vi "AuMT8852B EDR Sensitivity Configuration.vi"(5 "Settings":T2={"Low frequency selection"=enum."Use low frequency", "Medium frequency selection"=enum."Use medium frequency", "High frequency selection"=enum."Use high frequency", "Low TX frequency"=2480.0, "Low RX frequency"=2402.0, "Medium TX frequency"=2402.0, "Medium RX frequency"=2441.0, "High TX frequency"=2402.0, "High RX frequency"=2480.0, "Threshold bit count"=0.1, "2DHx test packet"=enum."OFF", "3DHx test packet"=enum."OFF", "Hop selection"=enum."Test with hopping off and on", "Test TX power"=-70.0, "Packet count"=enum."TX", "Total test bit count"=0.1, "Use Dirty transmitter"=FALSE, "Symbol timing error (ppm)"=[-20, -20, 20, 20, 20, -20, -20, -20, -20, 20], "Frequency offset (kHz)"=[75.0, 14.0, -2.0, 1.0, 39.0, 0.0, -42.0, 74.0, -19.0, -75.0], "Threshold error limit (E-5)"=7, "Total test error limit (E-4)"=1} {"Frequency offset (kHz)" format="%.2f"; "Symbol timing error (ppm)" format="%.1f"; "Total test bit count" format="%.2f"; "Test TX power" format="%.1f"; "Threshold bit count" format="%.2f"}, 7 "Set/Get (Set)":enum16{"Set", "Get"}(ring), 8 "error in (no error)":errorcluster, 10 "Script (3)":i32=3, 11 "VISA session":refnum<visa-resource-name>) -> (0 "error out":errorcluster, 2 "error code":i32, 3 "VISA session out":refnum<visa-resource-name>, 4 "Settings out":T1={"Low frequency selection"=enum."Use low frequency", "Medium frequency selection"=enum."Use medium frequency", "High frequency selection"=enum."Use high frequency", "Low TX frequency"=2480.0, "Low RX frequency"=2402.0, "Medium TX frequency"=2402.0, "Medium RX frequency"=2441.0, "High TX frequency"=2402.0, "High RX frequency"=2480.0, "Threshold bit count"=0.1, "2DHx test packet"=enum."OFF", "3DHx test packet"=enum."OFF", "Hop selection"=enum."Test with hopping off and on", "Test TX power"=-70.0, "Packet count"=enum."TX", "Total test bit count"=0.1, "Use Dirty transmitter"=FALSE, "Symbol timing error (ppm)"=[-20.0, -20.0, 20.0, 20.0, 20.0, -20.0, -20.0, -20.0, -20.0, 20.0], "Frequency offset (kHz)"=[75.0, 14.0, -2.0, 1.0, 39.0, 0.0, -42.0, 74.0, -19.0, -75.0], "Threshold error limit (E-5)"=7, "Total test error limit (E-4)"=1} {"Frequency offset (kHz)" format="%.2f"; "Symbol timing error (ppm)" format="%.2f"; "Total test bit count" format="%.2f"; "Test TX power" format="%.1f"; "Threshold bit count" format="%.2f"})   [LabVIEW 2017]
doc: "Anritsu MT8852B Bluetooth Tester\n\nConfigures the instrument for the EDR Sensitivity test.\n\nINPUTS\nSet/Get - whether the values are being sent to or retrieved from the instrument.\nScript - which of the stored scripts (1-10) will be queried or configured. Scripts 1 and 2 are read-only.\nSettings - parameters of the test to be written.\n\nOUTPUTS\nSettings out - current parameters of the test."
uses:
  <instrlib>/aumt8852B/General/Utilities/MT8850 Test Parameters.ctl
  <instrlib>/aumt8852B/General/Utilities/MT8850 Frequency Units.ctl
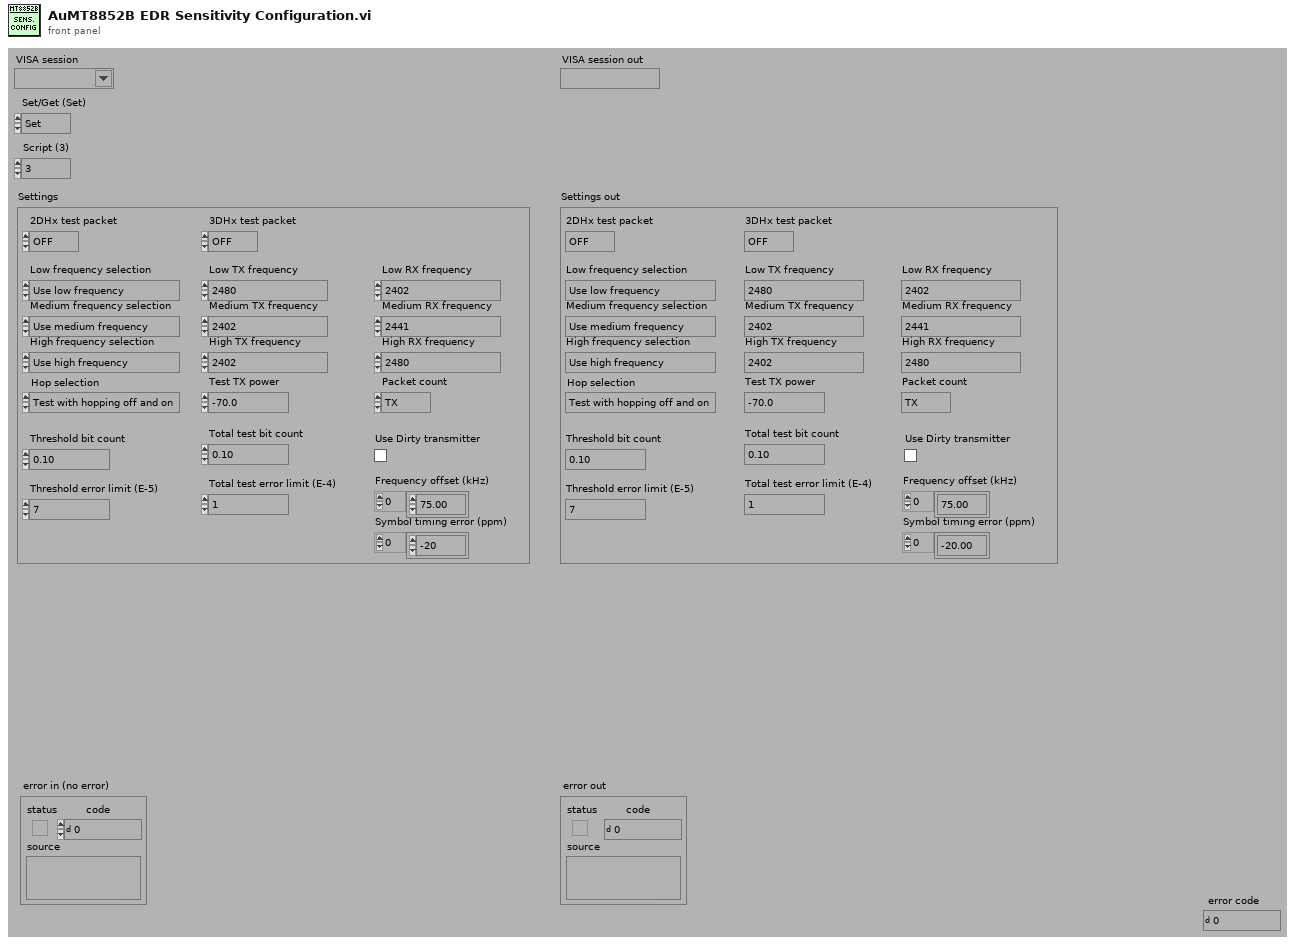
[diagram p1: front panel]
types:
  T1 = cluster{"Low frequency selection":enum16{"Don't use low frequency", "Use low frequency"}, "Medium frequency selection":enum16{"Don't use medium frequency", "Use medium frequency"}, "High frequency selection":enum16{"Don't use high frequency", "Use high frequency"}, "Low TX frequency":dbl, "Low RX frequency":dbl, "Medium TX frequency":dbl, "Medium RX frequency":dbl, "High TX frequency":dbl, "High RX frequency":dbl, "Threshold bit count":dbl, "2DHx test packet":enum16{"OFF", "Longest", "2-DH1", "2-DH3", "2-DH5"}, "3DHx test packet":enum16{"OFF", "Longest", "3-DH1", "3-DH3", "3-DH5"}, "Hop selection":enum16{"Test with hopping on", "Test with hopping off", "Test with hopping off and on"}, "Test TX power":dbl, "Packet count":enum16{"TX", "RX"}, "Total test bit count":dbl, "Use Dirty transmitter":bool, "Symbol timing error (ppm)":dbl[], "Frequency offset (kHz)":dbl[], "Threshold error limit (E-5)":i16, "Total test error limit (E-4)":i16}
  T2 = cluster{"Low frequency selection":enum16{"Don't use low frequency", "Use low frequency"}, "Medium frequency selection":enum16{"Don't use medium frequency", "Use medium frequency"}, "High frequency selection":enum16{"Don't use high frequency", "Use high frequency"}, "Low TX frequency":dbl, "Low RX frequency":dbl, "Medium TX frequency":dbl, "Medium RX frequency":dbl, "High TX frequency":dbl, "High RX frequency":dbl, "Threshold bit count":dbl, "2DHx test packet":enum16{"OFF", "Longest", "2-DH1", "2-DH3", "2-DH5"}, "3DHx test packet":enum16{"OFF", "Longest", "3-DH1", "3-DH3", "3-DH5"}, "Hop selection":enum16{"Test with hopping on", "Test with hopping off", "Test with hopping off and on"}, "Test TX power":dbl, "Packet count":enum16{"TX", "RX"}, "Total test bit count":dbl, "Use Dirty transmitter":bool, "Symbol timing error (ppm)":i8[], "Frequency offset (kHz)":dbl[], "Threshold error limit (E-5)":i16, "Total test error limit (E-4)":i16}
  T3 = enum16{"Frequency offset", "Symbol timing value", "Mod index value"}
  T4 = enum16{"Single-slot sensitivity", "Multiple-slot sensitivity", "EDR sensitivity"}
  T5 = typedef "MT8850 Test Parameters.ctl" = enum16{"Use low frequency", "Use medium frequency", "Use high frequency", "Low TX frequency", "Low RX frquency", "Medium TX frequency", "Medium RX frequency", "High TX frequency", "High RX frequency", "Number of packets", "Average high limit", "Average low limit", "Peak power limit", "Max power step limit", "Min power step limit", "f1 average minimum", "f1 average maximum", "f2 maximum", "f1/f2 average maximum", "Hop selection", "Use DH1 packets", "Use DH3 packets", "Use DH5 packets", "1 slot packet drift limit", "3 slot packet drift limit", "5 slot packet drift limit", "Drift rate limit", "TX power level", "Frequency offset", "Symbol timing", "Modulation index", "BER limit", "FER limit", "Use averaging high limit", "Use averaging low limit", "Use peak power limit", "Packet type", "Test control", "Use max power step limit", "Use min power step limit", "Number of cycles", "Use f1 average maximum", "Use f1 average minimum", "Use f2 maximum", "Use f1/f2 average maximum", "Hop mode", "Maximum negative limit", "Maximum positive limit", "Use maximum negative limit", "Use maximum positive limit", "Use 1 slot packet drift limit", "Use 3 slot packet drift limit", "Use 5 slot packet drift limit", "Use drift rate limit", "Use BER limit", "Use FER limit", "Use dirty parameter table", "Use null packet drift limit", "Null packet drift limit", "Minimum power", "Power delay", "Packet count", "Payload toggle", "Output power level", "2DHX packet type", "3DHX packet type", "Number of blocks", "TX and RX low frequency", "TX and RX medium frequency", "TX and RX high frequency", "TX frequency", "RX frequency", "Threshold bit count", "Total test bit count", "Number of bits", "PDPSK to PGFSK lower limit", "PDPSK to PGFSK upper limit", "Initial frequency error upper limit", "Initial frequency error lower limit", "Frequency error upper limit", "Frequency error lower limit", "Block frequency error upper limit", "Block frequency error lower limit", "2Mbs RMS DEVM limit", "3Mbs RMS DEVM limit", "2Mbs Peak DEVM limit", "3Mbs Peak DEVM limit", "2Mbs 99% packets DEVM limit", "3Mbs 99% packets DEVM limit", "Percentage of no error packets limit", "Threshold error limit", "Total test error limit"}
  T6 = enum16{"Output power", "Power control", "Modulation characteristics", "Initial carrier", "Carrier drift", "Single slot sensitivity", "Multiple slot sensitivity", "Maximum input power", "EDR Relative transmit power", "EDR Carrier frequency and stability", "EDR Differential phase encoding", "EDR Sensitivity", "EDR BER floor sensitivity", "EDR Maximum input power"}
  T7 = typedef "MT8850 Frequency Units.ctl" = enum16{"Channel", "Hz", "kHz", "MHz", "GHz"}
  T8 = enum16{"Simulate", "Range check", "Cache", "Query instrument status"}
  T9 = enum16{"Test with hopping on", "Test with hopping off", "Test with hopping off and on"}
  T10 = enum16{"OFF", "Longest", "3-DH1", "3-DH3", "3-DH5"}
  T11 = enum16{"OFF", "Longest", "2-DH1", "2-DH3", "2-DH5"}
  T12 = enum16{"Don't use high frequency", "Use high frequency"}
  T13 = enum16{"Don't use medium frequency", "Use medium frequency"}
  T14 = enum16{"Don't use low frequency", "Use low frequency"}
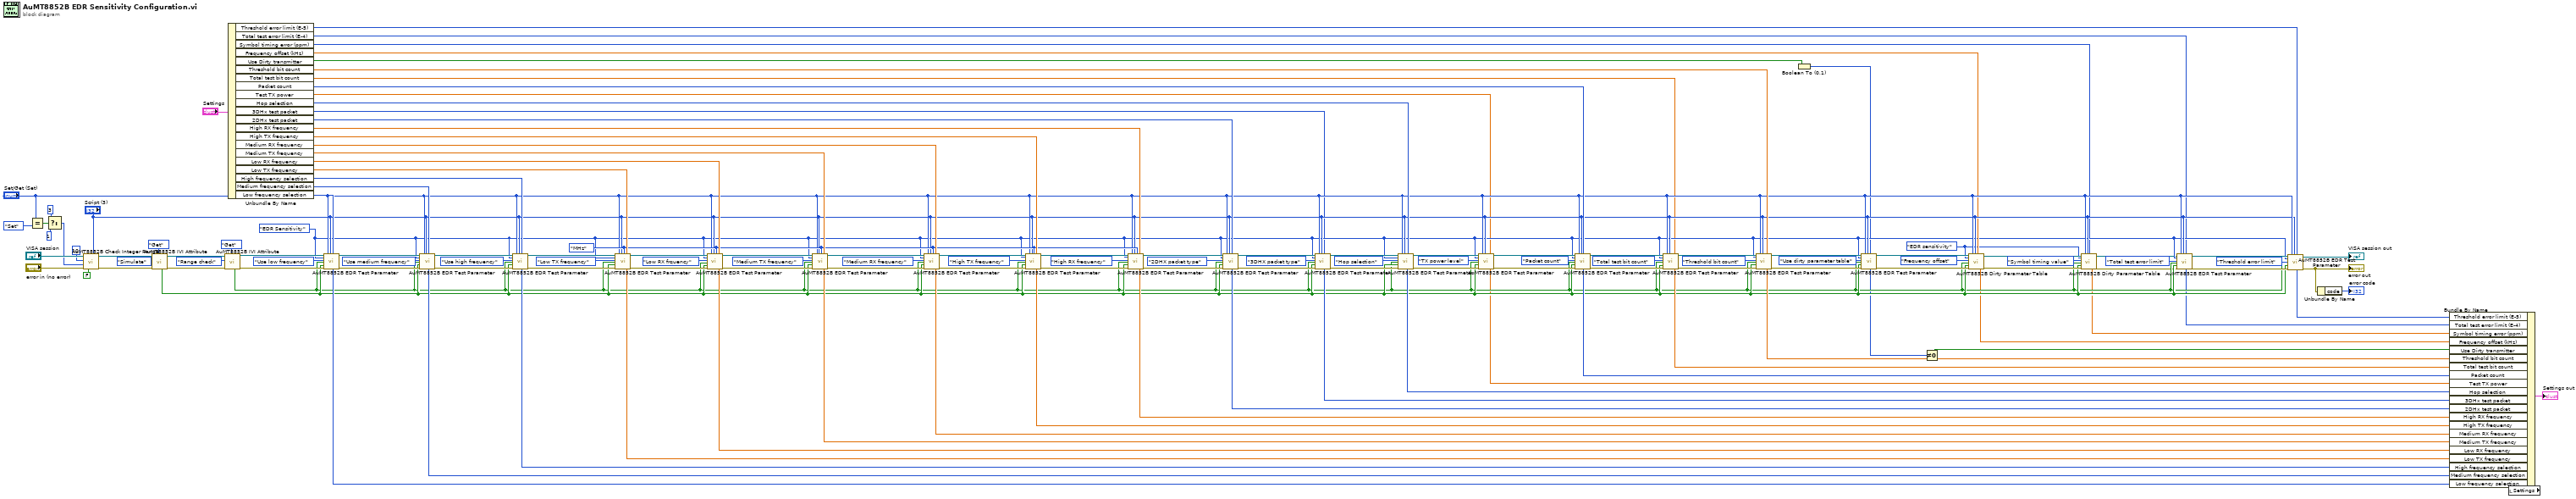
[diagram p0: block diagram]
diagram:
  w14 = T4."EDR sensitivity" ("Test (Single-slot sensitivity)")
  w15 = T6."EDR Sensitivity" ("Test (Output power)")
  w65 = MT8850_Frequency_Units."MHz" ("Frequency units (MHz)")
  n1 = Equal?(x="Set/Get (Set)", y=enum16{"Set", "Get"}."Set") -> (x = y?=w134:bool)
  n2 = Select(t=3, s=w134, f=1) -> (s? t:f=w130:i32)
  n3 = call <instrlib>:"AuMT8852B Check Integer Range.vi"("Value (0)"="Script (3)", "Check IVI flag first? (T)"=FALSE, "error in (no error)"="error in (no error)", "Lower limit (-1)"=w130, "Upper limit (1)"=10, "VISA session"="VISA session") -> ("error out"=w128:errorcluster, "VISA session out"=w129:refnum<visa-resource-name>)  [unwired: 4 in]
  n4 = call <instrlib>:"AuMT8852B IVI Attribute.vi"("Set/Get (Set)"=enum16{"Set", "Get"}."Get", "error in (no error)"=w128, "Flag (Simulate)"=T8."Simulate", "VISA session"=w129) -> ("error out"=w102:errorcluster, "VISA session out"=w103:refnum<visa-resource-name>, "Value out"=w30:bool)  [unwired: 5 in]
  n5 = call <instrlib>:"AuMT8852B IVI Attribute.vi"("Set/Get (Set)"=enum16{"Set", "Get"}."Get", "error in (no error)"=w102, "Flag (Simulate)"=T8."Range check", "VISA session"=w103) -> ("error out"=w100:errorcluster, "VISA session out"=w101:refnum<visa-resource-name>, "Value out"=w29:bool)  [unwired: 5 in]
  n6 = Unbundle By Name("Settings") -> ("Threshold error limit (E-5)"=w2:i16, "Total test error limit (E-4)"=w3:i16, "Symbol timing error (ppm)"=w11:i8[], "Frequency offset (kHz)"=w17:dbl[], "Use Dirty transmitter"=w19:bool, "Threshold bit count"=w35:dbl, "Total test bit count"=w7:dbl, "Packet count"=w50:enum16{"TX", "RX"}, "Test TX power"=w1:dbl, "Hop selection"=w56:T9, "3DHx test packet"=w8:T10, "2DHx test packet"=w78:T11, "High RX frequency"=w90:dbl, "High TX frequency"=w91:dbl, "Medium RX frequency"=w79:dbl, "Medium TX frequency"=w92:dbl, "Low RX frequency"=w93:dbl, "Low TX frequency"=w94:dbl, "High frequency selection"=w95:T12, "Medium frequency selection"=w96:T13, "Low frequency selection"=w97:T14)
  n7 = call <instrlib>:"AuMT8852B EDR Test Parameter.vi"("VISA session"=w101, "Test (Output power)"=w15, "Parameter (Use low frequency)"=MT8850_Test_Parameters."Use low frequency", "Range check? (F)"=w29, "Simulate? (F)"=w30, "error in (no error)"=w100, "Set/Get (Set)"="Set/Get (Set)", "Script (3)"="Script (3)", "Integer value (0)"=w97) -> ("Integer value out"=w82:i32, "VISA session out"=w71:refnum<visa-resource-name>, "error out"=w70:errorcluster)  [unwired: 7 in, 1 out]
  n8 = call <instrlib>:"AuMT8852B EDR Test Parameter.vi"("VISA session"=w71, "Test (Output power)"=w15, "Parameter (Use low frequency)"=MT8850_Test_Parameters."Use medium frequency", "Range check? (F)"=w29, "Simulate? (F)"=w30, "error in (no error)"=w70, "Set/Get (Set)"="Set/Get (Set)", "Script (3)"="Script (3)", "Integer value (0)"=w96) -> ("Integer value out"=w83:i32, "VISA session out"=w69:refnum<visa-resource-name>, "error out"=w68:errorcluster)  [unwired: 7 in, 1 out]
  n9 = call <instrlib>:"AuMT8852B EDR Test Parameter.vi"("VISA session"=w69, "Test (Output power)"=w15, "Parameter (Use low frequency)"=MT8850_Test_Parameters."Use high frequency", "Range check? (F)"=w29, "Simulate? (F)"=w30, "error in (no error)"=w68, "Set/Get (Set)"="Set/Get (Set)", "Script (3)"="Script (3)", "Integer value (0)"=w95) -> ("Integer value out"=w84:i32, "VISA session out"=w124:refnum<visa-resource-name>, "error out"=w123:errorcluster)  [unwired: 7 in, 1 out]
  n10 = call <instrlib>:"AuMT8852B EDR Test Parameter.vi"("VISA session"=w124, "Test (Output power)"=w15, "Parameter (Use low frequency)"=MT8850_Test_Parameters."Low TX frequency", "Range check? (F)"=w29, "Simulate? (F)"=w30, "error in (no error)"=w123, "Set/Get (Set)"="Set/Get (Set)", "Script (3)"="Script (3)", "Integer value (0)"=w65, "Float value (0)"=w94) -> ("Float value out"=w85:dbl, "VISA session out"=w122:refnum<visa-resource-name>, "error out"=w121:errorcluster)  [unwired: 6 in, 1 out]
  n11 = call <instrlib>:"AuMT8852B EDR Test Parameter.vi"("VISA session"=w122, "Test (Output power)"=w15, "Parameter (Use low frequency)"=MT8850_Test_Parameters."Low RX frquency", "Range check? (F)"=w29, "Simulate? (F)"=w30, "error in (no error)"=w121, "Set/Get (Set)"="Set/Get (Set)", "Script (3)"="Script (3)", "Integer value (0)"=w65, "Float value (0)"=w93) -> ("Float value out"=w86:dbl, "VISA session out"=w120:refnum<visa-resource-name>, "error out"=w119:errorcluster)  [unwired: 6 in, 1 out]
  n12 = call <instrlib>:"AuMT8852B EDR Test Parameter.vi"("VISA session"=w120, "Test (Output power)"=w15, "Parameter (Use low frequency)"=MT8850_Test_Parameters."Medium TX frequency", "Range check? (F)"=w29, "Simulate? (F)"=w30, "error in (no error)"=w119, "Set/Get (Set)"="Set/Get (Set)", "Script (3)"="Script (3)", "Integer value (0)"=w65, "Float value (0)"=w92) -> ("Float value out"=w87:dbl, "VISA session out"=w118:refnum<visa-resource-name>, "error out"=w117:errorcluster)  [unwired: 6 in, 1 out]
  n13 = call <instrlib>:"AuMT8852B EDR Test Parameter.vi"("VISA session"=w118, "Test (Output power)"=w15, "Parameter (Use low frequency)"=MT8850_Test_Parameters."Medium RX frequency", "Range check? (F)"=w29, "Simulate? (F)"=w30, "error in (no error)"=w117, "Set/Get (Set)"="Set/Get (Set)", "Script (3)"="Script (3)", "Integer value (0)"=w65, "Float value (0)"=w79) -> ("Float value out"=w81:dbl, "VISA session out"=w116:refnum<visa-resource-name>, "error out"=w115:errorcluster)  [unwired: 6 in, 1 out]
  n14 = call <instrlib>:"AuMT8852B EDR Test Parameter.vi"("VISA session"=w116, "Test (Output power)"=w15, "Parameter (Use low frequency)"=MT8850_Test_Parameters."High TX frequency", "Range check? (F)"=w29, "Simulate? (F)"=w30, "error in (no error)"=w115, "Set/Get (Set)"="Set/Get (Set)", "Script (3)"="Script (3)", "Integer value (0)"=w65, "Float value (0)"=w91) -> ("Float value out"=w88:dbl, "VISA session out"=w114:refnum<visa-resource-name>, "error out"=w113:errorcluster)  [unwired: 6 in, 1 out]
  n15 = call <instrlib>:"AuMT8852B EDR Test Parameter.vi"("VISA session"=w114, "Test (Output power)"=w15, "Parameter (Use low frequency)"=MT8850_Test_Parameters."High RX frequency", "Range check? (F)"=w29, "Simulate? (F)"=w30, "error in (no error)"=w113, "Set/Get (Set)"="Set/Get (Set)", "Script (3)"="Script (3)", "Integer value (0)"=w65, "Float value (0)"=w90) -> ("Float value out"=w89:dbl, "VISA session out"=w112:refnum<visa-resource-name>, "error out"=w111:errorcluster)  [unwired: 6 in, 1 out]
  n16 = call <instrlib>:"AuMT8852B EDR Test Parameter.vi"("VISA session"=w112, "Test (Output power)"=w15, "Parameter (Use low frequency)"=MT8850_Test_Parameters."2DHX packet type", "Range check? (F)"=w29, "Simulate? (F)"=w30, "error in (no error)"=w111, "Set/Get (Set)"="Set/Get (Set)", "Script (3)"="Script (3)", "Integer value (0)"=w78) -> ("Integer value out"=w80:i32, "VISA session out"=w74:refnum<visa-resource-name>, "error out"=w73:errorcluster)  [unwired: 7 in, 1 out]
  n17 = call <instrlib>:"AuMT8852B EDR Test Parameter.vi"("VISA session"=w74, "Test (Output power)"=w15, "Parameter (Use low frequency)"=MT8850_Test_Parameters."3DHX packet type", "Range check? (F)"=w29, "Simulate? (F)"=w30, "error in (no error)"=w73, "Set/Get (Set)"="Set/Get (Set)", "Script (3)"="Script (3)", "Integer value (0)"=w8) -> ("Integer value out"=w49:i32, "VISA session out"=w59:refnum<visa-resource-name>, "error out"=w60:errorcluster)  [unwired: 7 in, 1 out]
  n18 = call <instrlib>:"AuMT8852B EDR Test Parameter.vi"("VISA session"=w59, "Test (Output power)"=w15, "Parameter (Use low frequency)"=MT8850_Test_Parameters."Hop selection", "Range check? (F)"=w29, "Simulate? (F)"=w30, "error in (no error)"=w60, "Set/Get (Set)"="Set/Get (Set)", "Script (3)"="Script (3)", "Integer value (0)"=w56) -> ("Integer value out"=w48:i32, "VISA session out"=w58:refnum<visa-resource-name>, "error out"=w61:errorcluster)  [unwired: 7 in, 1 out]
  n19 = call <instrlib>:"AuMT8852B EDR Test Parameter.vi"("VISA session"=w58, "Test (Output power)"=w15, "Parameter (Use low frequency)"=MT8850_Test_Parameters."TX power level", "Range check? (F)"=w29, "Simulate? (F)"=w30, "error in (no error)"=w61, "Set/Get (Set)"="Set/Get (Set)", "Script (3)"="Script (3)", "Float value (0)"=w1) -> ("Float value out"=w12:dbl, "VISA session out"=w53:refnum<visa-resource-name>, "error out"=w55:errorcluster)  [unwired: 7 in, 1 out]
  n20 = call <instrlib>:"AuMT8852B EDR Test Parameter.vi"("VISA session"=w53, "Test (Output power)"=w15, "Parameter (Use low frequency)"=MT8850_Test_Parameters."Packet count", "Range check? (F)"=w29, "Simulate? (F)"=w30, "error in (no error)"=w55, "Set/Get (Set)"="Set/Get (Set)", "Script (3)"="Script (3)", "Integer value (0)"=w50) -> ("Integer value out"=w47:i32, "VISA session out"=w52:refnum<visa-resource-name>, "error out"=w54:errorcluster)  [unwired: 7 in, 1 out]
  n21 = call <instrlib>:"AuMT8852B EDR Test Parameter.vi"("VISA session"=w52, "Test (Output power)"=w15, "Parameter (Use low frequency)"=MT8850_Test_Parameters."Total test bit count", "Range check? (F)"=w29, "Simulate? (F)"=w30, "error in (no error)"=w54, "Set/Get (Set)"="Set/Get (Set)", "Script (3)"="Script (3)", "Float value (0)"=w7) -> ("Float value out"=w34:dbl, "VISA session out"=w64:refnum<visa-resource-name>, "error out"=w63:errorcluster)  [unwired: 7 in, 1 out]
  n22 = call <instrlib>:"AuMT8852B EDR Test Parameter.vi"("VISA session"=w64, "Test (Output power)"=w15, "Parameter (Use low frequency)"=MT8850_Test_Parameters."Threshold bit count", "Range check? (F)"=w29, "Simulate? (F)"=w30, "error in (no error)"=w63, "Set/Get (Set)"="Set/Get (Set)", "Script (3)"="Script (3)", "Float value (0)"=w35) -> ("Float value out"=w33:dbl, "VISA session out"=w44:refnum<visa-resource-name>, "error out"=w46:errorcluster)  [unwired: 7 in, 1 out]
  n23 = Boolean To (0,1)(Boolean=w19) -> (0, 1=w6:i16)
  n24 = call <instrlib>:"AuMT8852B EDR Test Parameter.vi"("VISA session"=w44, "Test (Output power)"=w15, "Parameter (Use low frequency)"=MT8850_Test_Parameters."Use dirty parameter table", "Range check? (F)"=w29, "Simulate? (F)"=w30, "error in (no error)"=w46, "Set/Get (Set)"="Set/Get (Set)", "Script (3)"="Script (3)", "Integer value (0)"=w6) -> ("Integer value out"=w18:i32, "VISA session out"=w43:refnum<visa-resource-name>, "error out"=w45:errorcluster)  [unwired: 7 in, 1 out]
  n25 = Not Equal To 0?(x=w18) -> (x != 0?=w24:bool)
  n26 = call <instrlib>:"AuMT8852B Dirty Parameter Table.vi"("VISA session"=w43, "Test (Single-slot sensitivity)"=w14, "Variable (Frequency offset)"=T3."Frequency offset", "Range check? (F)"=w29, "Simulate? (F)"=w30, "error in (no error)"=w45, "Set/Get (Set)"="Set/Get (Set)", "Script (3)"="Script (3)", "Parameters"=w17) -> ("Parameters out"=w21:dbl[], "VISA session out"=w27:refnum<visa-resource-name>, "error out"=w38:errorcluster)  [unwired: 8 in]
  n27 = call <instrlib>:"AuMT8852B Dirty Parameter Table.vi"("VISA session"=w27, "Test (Single-slot sensitivity)"=w14, "Variable (Frequency offset)"=T3."Symbol timing value", "Range check? (F)"=w29, "Simulate? (F)"=w30, "error in (no error)"=w38, "Set/Get (Set)"="Set/Get (Set)", "Script (3)"="Script (3)", "Parameters"=w11) -> ("Parameters out"=w20:dbl[], "VISA session out"=w9:refnum<visa-resource-name>, "error out"=w10:errorcluster)  [unwired: 8 in]
  n28 = call <instrlib>:"AuMT8852B EDR Test Parameter.vi"("VISA session"=w9, "Test (Output power)"=w15, "Parameter (Use low frequency)"=MT8850_Test_Parameters."Total test error limit", "Range check? (F)"=w29, "Simulate? (F)"=w30, "error in (no error)"=w10, "Set/Get (Set)"="Set/Get (Set)", "Script (3)"="Script (3)", "Integer value (0)"=w3) -> ("Integer value out"=w4:i32, "VISA session out"=w28:refnum<visa-resource-name>, "error out"=w37:errorcluster)  [unwired: 7 in, 1 out]
  n29 = call <instrlib>:"AuMT8852B EDR Test Parameter.vi"("VISA session"=w28, "Test (Output power)"=w15, "Parameter (Use low frequency)"=MT8850_Test_Parameters."Threshold error limit", "Range check? (F)"=w29, "Simulate? (F)"=w30, "error in (no error)"=w37, "Set/Get (Set)"="Set/Get (Set)", "Script (3)"="Script (3)", "Integer value (0)"=w2) -> ("Integer value out"=w5:i32, "VISA session out"=→"VISA session out":refnum<visa-resource-name>, "error out"=w23:errorcluster)  [unwired: 7 in, 1 out]
  "error out" <- w23
  n30 = Unbundle By Name(w23) -> ("code"=→"error code":i32)
  n31 = local read "Settings"() -> (w40:T2)
  n32 = Bundle By Name(cluster=w40, "Threshold error limit (E-5)"=w5, "Total test error limit (E-4)"=w4, "Symbol timing error (ppm)"=w20, "Frequency offset (kHz)"=w21, "Use Dirty transmitter"=w24, "Threshold bit count"=w33, "Total test bit count"=w34, "Packet count"=w47, "Test TX power"=w12, "Hop selection"=w48, "3DHx test packet"=w49, "2DHx test packet"=w80, "High RX frequency"=w89, "High TX frequency"=w88, "Medium RX frequency"=w81, "Medium TX frequency"=w87, "Low RX frequency"=w86, "Low TX frequency"=w85, "High frequency selection"=w84, "Medium frequency selection"=w83, "Low frequency selection"=w82) -> (→"Settings out":T2)
